vi "Test Leakage.vi"(11 "VISA Refnum in":refnum<visa-resource-name>) -> (0 "error out":errorcluster, 2 "BoardHandle out":T1)   [LabVIEW 2020]
uses:
  Program Files/National Instruments/LabVIEW 2018/instr.lib/CAEN PSM/CAEN PSM.lvlib
panel:
  # "DO NOT RUN THIS WHEN TUBES ARE IN"
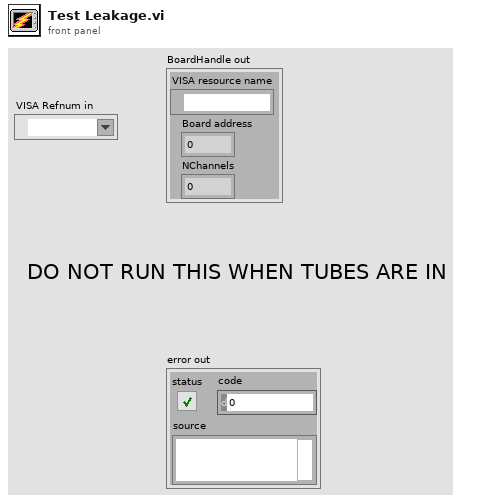
[diagram p1: front panel]
types:
  T1 = cluster{"VISA resource name":refnum<visa-resource-name>, "Board address":u8, "NChannels":u8}
  T2 = typedef "CAEN PSM.lvlib/BoardHandle.ctl" = cluster{"VISA resource name":refnum<visa-resource-name>, "Board address":u8, "NChannels":u8}
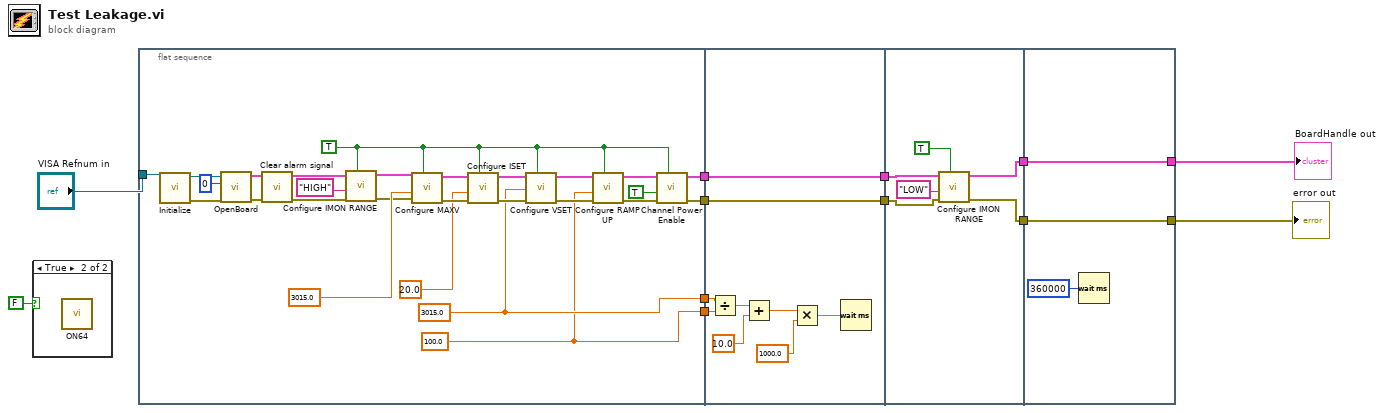
[diagram p0: block diagram]
diagram:
  n1 = case shown="True" FALSE {
    frame False {
    }
    frame True {
      n2 = call "ON64.vi"() -> ()  [unwired: 2 in]
    }
  }
  n3 = flat-sequence {
    tunnel: [w25] -> w12
    tunnel: [w24] -> w11
    tunnel: [w23] -> w10
    tunnel: [w22] -> w9
    tunnel: "VISA Refnum in" -> [w21]
    tunnel: w12 -> [w43]
    tunnel: w11 -> [w42]
    tunnel: w10 -> [w41]
    tunnel: w9 -> [w40]
    tunnel: [w41] -> w7
    tunnel: [w40] -> w6
    tunnel: w7 -> [w52]
    tunnel: w6 -> [w51]
    tunnel: [w50] -> w3
    tunnel: [w49] -> w2
    tunnel: [w56] -> w4
    tunnel: [w57] -> w5
    tunnel: w3 -> [w57]
    tunnel: w2 -> [w56]
    frame #0 {
      w14 = TRUE ("All Channels (F)")
      w25 = 3015.0 ("Voltage Set (Volts)")
      w24 = 100.0 ("Voltage Ramp Up (V/s)")
      n4 = call "Initialize.vi"("VISA resource name"=w21) -> ("error out"=w34:errorcluster, "VISA resource name out"=w31:refnum<visa-resource-name>)  [unwired: 9 in]
      n5 = call "OpenBoard.vi"("error in (no error)"=w34, "Board Address"=u8 0, "VISA resource name"=w31) -> ("error out"=w35:errorcluster, "BoardHandle"=w30:T2)  [unwired: 7 in]
      n6 = call "Clear alarm signal.vi"("error in (no error)"=w35, "BoardHandle"=w30) -> ("error out"=w19:errorcluster, "BoardHandle out"=w18:T2)  [unwired: 8 in]
      n7 = call "Configure IMON RANGE.vi"("All Channels (F)"=w14, "error in (no error)"=w19, "IMon range (LOW)"="HIGH", "BoardHandle"=w18) -> ("error out"=w15:errorcluster, "BoardHandle out"=w16:T2)  [unwired: 6 in]
      n8 = call "Configure MAXV.vi"("All Channels (F)"=w14, "error in (no error)"=w15, "Voltage Max (0.0 V)"=3015.0 ("VMax (Volts)"), "BoardHandle"=w16) -> ("error out"=w36:errorcluster, "BoardHandle out"=w29:T2)  [unwired: 6 in]
      n9 = call "Configure ISET.vi"("All Channels (F)"=w14, "error in (no error)"=w36, "Current Limit (0.00 uA)"=20.0 ("Current Limit (uA)"), "BoardHandle"=w29) -> ("error out"=w37:errorcluster, "BoardHandle out"=w28:T2)  [unwired: 6 in]
      n10 = call "Configure VSET.vi"("All Channels (F)"=w14, "error in (no error)"=w37, "Voltage Level (0.0 V)"=w25, "BoardHandle"=w28) -> ("error out"=w38:errorcluster, "BoardHandle out"=w27:T2)  [unwired: 6 in]
      n11 = call "Configure RAMP UP.vi"("All Channels (F)"=w14, "error in (no error)"=w38, "Voltage ramp up (0 V/s)"=w24, "BoardHandle"=w27) -> ("error out"=w39:errorcluster, "BoardHandle out"=w26:T2)  [unwired: 6 in]
      n12 = call "Channel Power Enable.vi"("All Channels (F)"=w14, "error in (no error)"=w39, "Enable (OFF)"=TRUE ("Boolean"), "BoardHandle"=w26) -> ("error out"=w22:errorcluster, "BoardHandle out"=w23:T2)  [unwired: 6 in]
    }
    frame #1 {
      n13 = Divide(x=w43, y=w42) -> (x/y=w46:dbl)
      n14 = Add(x=w46, y=10.0) -> (x+y=w47:dbl)
      n15 = Multiply(x=w47, y=1000.0) -> (x*y=w48:dbl)
      n16 = Wait (ms)(milliseconds to wait=w48) -> ()  [unwired: 1 out]
    }
    frame #2 {
      n17 = call "Configure IMON RANGE.vi"("All Channels (F)"=TRUE, "error in (no error)"=w51, "IMon range (LOW)"="LOW", "BoardHandle"=w52) -> ("error out"=w50:errorcluster, "BoardHandle out"=w49:T2)  [unwired: 6 in]
    }
    frame #3 {
      n18 = Wait (ms)(milliseconds to wait=u32 360000) -> ()  [unwired: 1 out]
    }
  }
  "BoardHandle out" <- w4
  "error out" <- w5
